vi "plant.vi"(8 "error in (no error)":errorcluster, 11 "Dynamic-System in":refnum<class "Dynamic-System.lvclass">) -> (0 "error out":errorcluster, 1 "End of Simulation?":bool, 2 "output cluster":cluster{"Time":dbl[], "State 1":dbl[]}, 3 "Dynamic-System out":refnum<class "Dynamic-System.lvclass">, 4 "% Complete":u8)   [LabVIEW 2025, in "Dynamic-System.lvclass"]
uses:
  Dynamic-System.lvclass
  Dynamic-System.lvclass/Dynamic-System.ctl
  <vilib>/gmath/NI_Gmath.lvlib
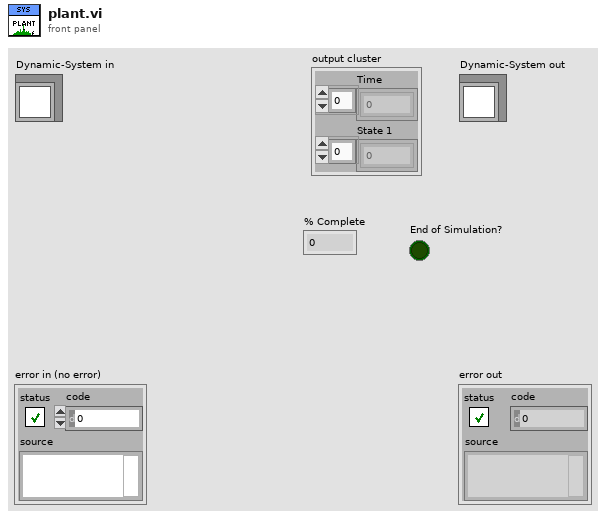
[diagram p1: front panel]
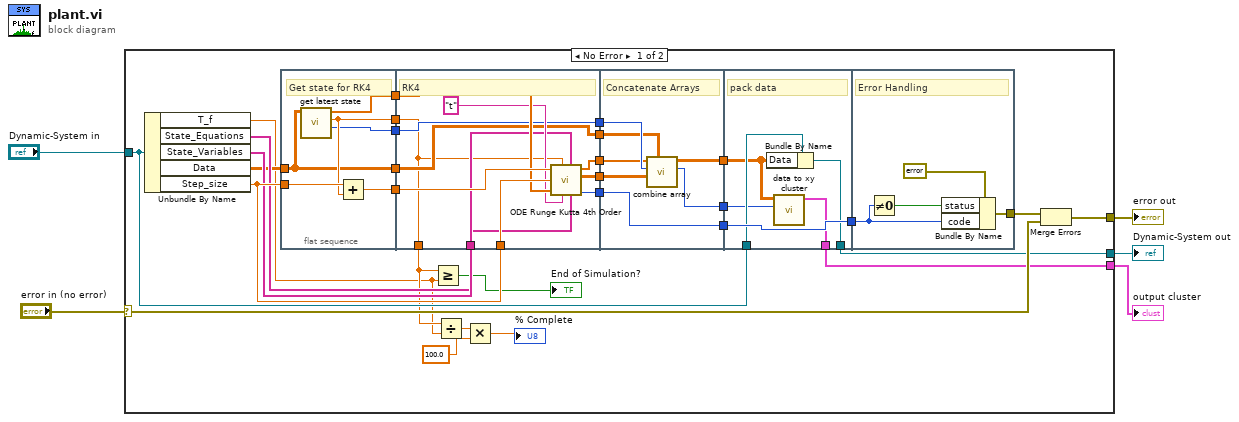
[diagram p0: block diagram]
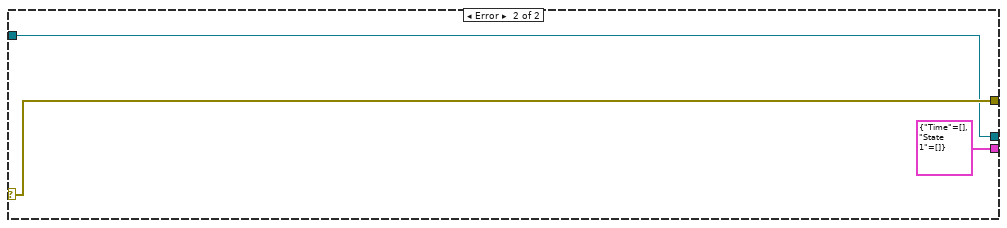
[diagram p2: hidden frame]
diagram:
  n1 = case shown="No Error" "error in (no error)" {
    selector: "error in (no error)" -> [w22 w73]
    tunnel: [w21 w73] -> w4
    tunnel: [w14 w72] -> w2
    tunnel: "Dynamic-System in" -> [w16 w72]
    tunnel: [w15 cluster{"Time":dbl[], "State 1":dbl[]} {"Time"=[], "State 1"=[]} ("input cluster")] -> w1
    frame No Error {
      n2 = Unbundle By Name(w16) -> ("T_f"=w9:dbl, "State_Equations"=w30:string[], "State_Variables"=w31:string[], "Data"=w27:dbl[][], "Step_size"=w32:dbl)
      n3 = flat-sequence {
        tunnel: w32 -> [w41]
        tunnel: w27 -> [w36]
        tunnel: [w40] -> w35
        tunnel: [w39] -> w34
        tunnel: [w38] -> w33
        tunnel: [w37] -> w26
        tunnel: [w36] -> w20
        tunnel: w35 -> [w42]
        tunnel: w34 -> [w53]
        tunnel: w33 -> [w51]
        tunnel: w32 -> [w52]
        tunnel: w31 -> [w49]
        tunnel: w30 -> [w48]
        tunnel: [w47] -> w29
        tunnel: [w46] -> w28
        tunnel: w26 -> [w45]
        tunnel: [w45] -> w25
        tunnel: [w44] -> w24
        tunnel: w20 -> [w43]
        tunnel: [w43] -> w19
        tunnel: [w42] -> w10
        tunnel: w29 -> [w57]
        tunnel: w28 -> [w59]
        tunnel: w25 -> [w58]
        tunnel: w24 -> [w60]
        tunnel: [w60] -> w18
        tunnel: w19 -> [w56]
        tunnel: [w55] -> w13
        tunnel: [w54] -> w12
        tunnel: w18 -> [w66]
        tunnel: [w66] -> w17
        tunnel: w16 -> [w65]
        tunnel: [w64] -> w15
        tunnel: [w63] -> w14
        tunnel: w13 -> [w62]
        tunnel: w12 -> [w61]
        tunnel: w17 -> [w68]
        tunnel: [w67] -> w23
        frame #0 {
          # "Get state for RK4"
          n4 = call "get latest state.vi"("t & X"=w36) -> ("end element"=w37:i32, "Time [s]"=w40:dbl, "X_i"=w38:dbl[])  [unwired: 8 in]
          n5 = Add(x=w41, y=w40) -> (x+y=w39:dbl)
        }
        frame #1 {
          # "RK4"
          n6 = call <vilib>:"ODE Runge Kutta 4th Order.vi"("time end"=w53, "time start"=w42, "h (step rate)"=w52, "X0"=w51, "time"="t", "X (name of variables)"=w49, "F(X,t) (right sides of the ODE\nas functions of X and t)"=w48) -> ("Times"=w47:dbl[], "X Values (solution)"=w46:dbl[][], "error"=w44:i32)  [unwired: 1 out]
        }
        frame #2 {
          # "Concatenate Arrays"
          n7 = call "combine array.vi"("Previous Data"=w56, "X Values (solution)"=w59, "end element"=w58, "Times in"=w57) -> ("Index"=w54:i32, "Combined Data"=w55:dbl[][])  [unwired: 6 in]
        }
        frame #3 {
          # "pack data"
          n8 = Bundle By Name(cluster=w65, "Data"=w62) -> (w63:refnum<class "Dynamic-System.lvclass">)
          n9 = call "data to xy cluster.vi"("Index"=w61, "Combined Data"=w62) -> ("input cluster"=w64:cluster{"Time":dbl[], "State 1":dbl[]})  [unwired: 9 in]
        }
        frame #4 {
          # "Error Handling"
          n10 = Not Equal To 0?(x=w68) -> (x != 0?=w69:bool)
          n11 = Bundle By Name(cluster=errorcluster {"status"=FALSE, "code"=0, "source"=""} ("error constant"), "status"=w69, "code"=w68) -> (w67:errorcluster)
        }
      }
      n12 = Greater Or Equal?(x=w10, y=w9) -> (x >= y?=→"End of Simulation?":bool)
      n13 = Divide(x=w10, y=w9) -> (x/y=w8:dbl)
      n14 = Multiply(x=w8, y=100.0) -> (x*y=→"% Complete":dbl)
      n15 = Merge Errors(w23, w22) -> (w21:errorcluster)
    }
    frame Error {
    }
  }
  "error out" <- w4
  "Dynamic-System out" <- w2
  "output cluster" <- w1
